vi "subsetupRxHWParameters.vi"(0 "IVI Refnum in":refnum<k15>, 5 "Rx Parameters":T1, 11 "error in (no error)":errorcluster) -> (4 "IVI Refnum out":refnum<k15>, 6 "Rx Parameters":T1, 15 "error out":errorcluster)   [LabVIEW 2015]
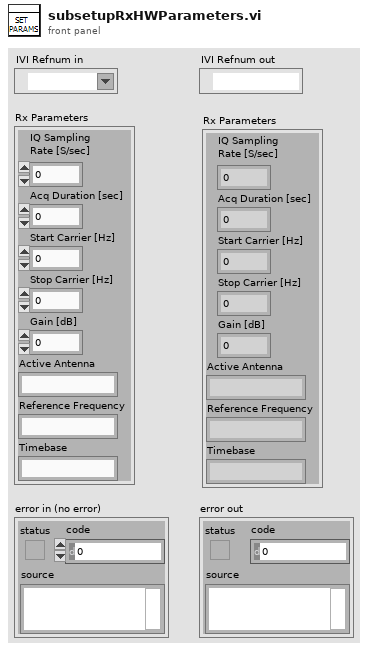
[diagram p1: front panel]
types:
  T1 = cluster{"IQ Sampling\nRate [S/sec]":dbl, "Acq Duration [sec]":dbl, "Start Carrier [Hz]":dbl, "Stop Carrier [Hz]":dbl, "Gain [dB]":dbl, "Active Antenna":string, "Reference Frequency":string, "Timebase":string}
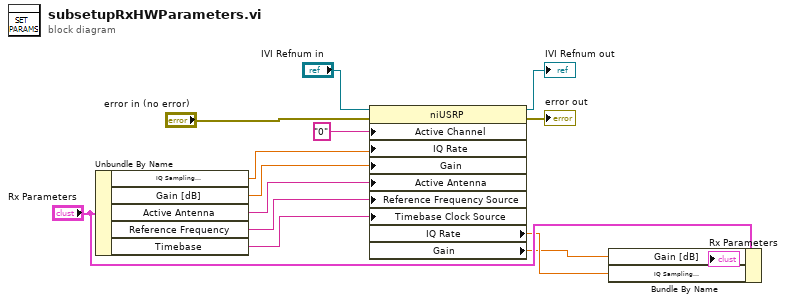
[diagram p0: block diagram]
diagram:
  n1 = Unbundle By Name("Rx Parameters") -> ("IQ Sampling\nRate [S/sec]"=w6:dbl, "Gain [dB]"=w7:dbl, "Active Antenna"=w8:string, "Reference Frequency"=w9:string, "Timebase"=w10:string)
  n2 = property class="niUSRP"(reference="IVI Refnum in", error in="error in (no error)", "Active Channel"="0", "IQ Rate"=w6, "Gain"=w7, "Active Antenna"=w8, "Reference Frequency Source"=w9, "Timebase Clock Source"=w10) -> (reference out=→"IVI Refnum out":refnum<k15>, error out=→"error out":errorcluster, "IQ Rate"=w4:dbl, "Gain"=w2:dbl)
  n3 = Bundle By Name(cluster="Rx Parameters", "Gain [dB]"=w2, "IQ Sampling\nRate [S/sec]"=w4) -> (→"Rx Parameters":T1)
